vi "Untitled 2.vi"() -> ()   [LabVIEW 2020]
panel:
  out "Dustbin Door":bool
  out "Human Detection":bool
  out "Dustbin Space":bool
  in  "VISA resource name":refnum<visa-resource-name>
  in  "Table Control":string[][](table)
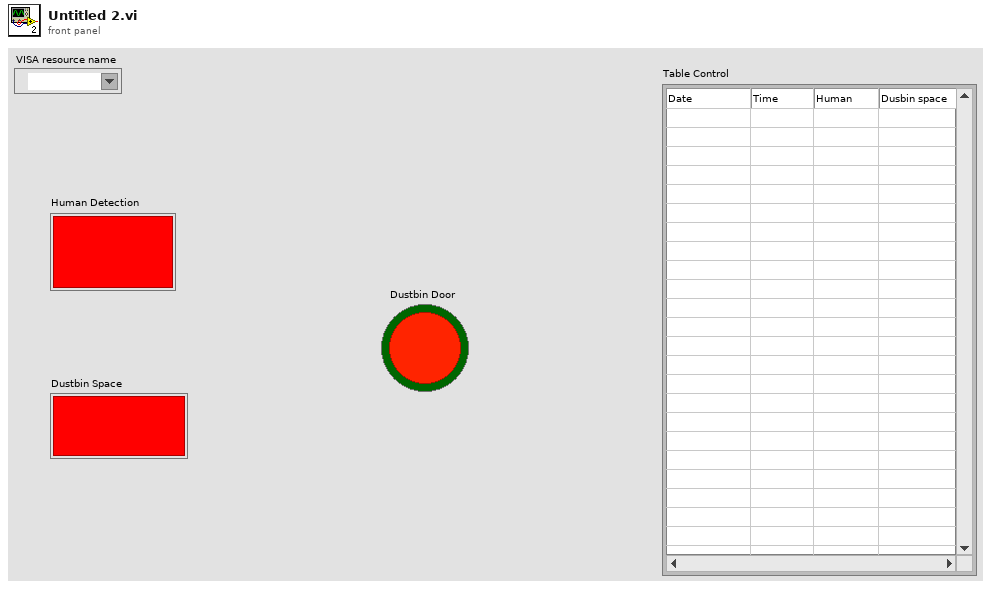
[diagram p1: front panel]
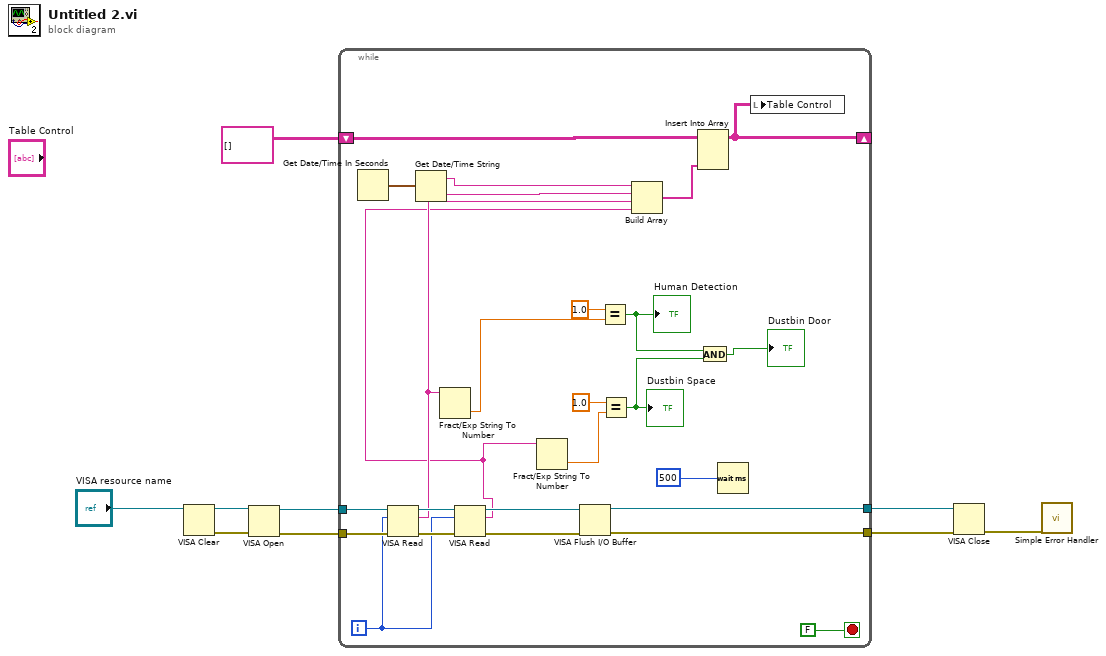
[diagram p0: block diagram]
diagram:
  n1 = VISA Clear(VISA resource name="VISA resource name") -> (VISA resource name out=w9:refnum<visa-resource-name>, error out=w8:errorcluster)  [unwired: 1 in]
  n2 = VISA Open(error in (no error)=w8, VISA resource name=w9) -> (VISA resource name=w7:refnum<visa-resource-name>, error out=w6:errorcluster)  [unwired: 3 in]
  n3 = while {
    tunnel: w7 -> [w35]
    tunnel: w6 -> [w34]
    tunnel: [w29] -> w5
    tunnel: [w28] -> w4
    shift-right: [w24] -> _
    shift-left: string[][] [] -> [w25]
    i -> [w27]
    stop <- FALSE stop-if-true
    n4 = Get Date/Time In Seconds() -> (seconds since 1Jan1904=w23:timestamp)
    n5 = VISA Read(VISA resource name=w35, byte count=w27, error in (no error)=w34) -> (VISA resource name out=w33:refnum<visa-resource-name>, read buffer=w20:string, error out=w32:errorcluster)  [unwired: 1 out]
    n6 = Get Date/Time String(seconds (now)=w23) -> (date string=w22:string, time string=w21:string)  [unwired: 2 in]
    n7 = Fract/Exp String To Number(string=w20) -> (number=w16:dbl)  [unwired: 3 in, 1 out]
    n8 = VISA Read(VISA resource name=w33, byte count=w27, error in (no error)=w32) -> (VISA resource name out=w31:refnum<visa-resource-name>, read buffer=w19:string, error out=w30:errorcluster)  [unwired: 1 out]
    n9 = Fract/Exp String To Number(string=w19) -> (number=w10:dbl)  [unwired: 3 in, 1 out]
    n10 = VISA Flush I/O Buffer(VISA resource name=w31, error in (no error)=w30) -> (VISA resource name out=w29:refnum<visa-resource-name>, error out=w28:errorcluster)  [unwired: 1 in]
    n11 = Equal?(x=1.0, y=w16) -> (x = y?=w13:bool)
    "Human Detection" <- w13
    n12 = Equal?(x=1.0, y=w10) -> (x = y?=w12:bool)
    "Dustbin Space" <- w12
    n13 = Build Array(w22, w21, w20, w19) -> (w17:string[])
    n14 = Insert Into Array(array=w25, new element=w17) -> (w24:string[][])  [unwired: 2 in]
    n15 = And(x=w13, y=w12) -> (x .and. y?=→"Dustbin Door":bool)
    n16 = Wait (ms)(milliseconds to wait=u32 500 ("millisecond timer value")) -> ()  [unwired: 1 out]
    n17 = local write "Table Control"(w24) -> ()
  }
  n18 = VISA Close(VISA resource name=w5, error in (no error)=w4) -> (error out=w3:errorcluster)
  n19 = call <vilib>:"Simple Error Handler.vi"("error in (no error)"=w3) -> ()  [unwired: 4 in, 5 out]
